vi "Nchw_CheckSize.vi"(4 "NumberOfMats":i32, 6 "MatToFit":T1, 8 "Width":i32, 9 "Height":i32, 10 "Channels":i32, 11 "Dimensions":i32) -> (3 "same":bool)   [LabVIEW 2020, in "OpenLvVision_OpenCv.lvlib"]
uses:
  OpenLvVision_OpenCv.lvlib
  TypeDef/LvDatatype.ctl
  TypeDef/MatInfo.ctl
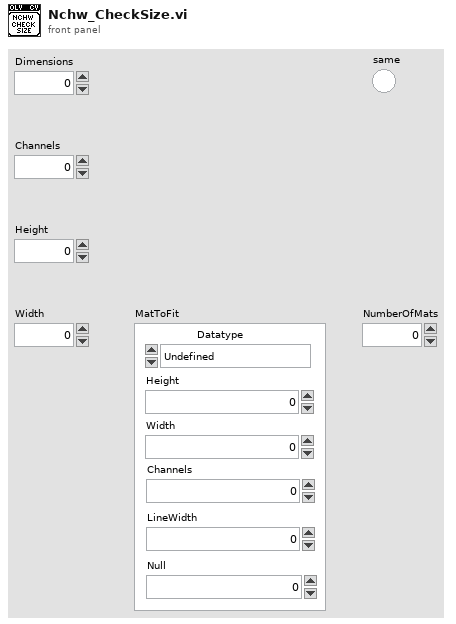
[diagram p1: front panel]
types:
  T1 = typedef "OpenLvVision_OpenCv.lvlib/MatInfo.ctl" = cluster{"Datatype":T2, "Height":i32, "Width":i32, "Channels":i32, "LineWidth":i32, "Null":u8}
  T2 = typedef "OpenLvVision_OpenCv.lvlib/LvDatatype.ctl" = enum32{"Undefined", "U8", "I8", "U16", "I16", "U32_Color", "I32", "U64_Color", "I64", "SGL", "DBL", "Complex SGL", "Complex DBL", "Array 1D U8", "Array 1D I8", "Array 1D U16", "Array 1D I16", "Array 1D U32_Color", "Array 1D I32", "Array 1D U64_Color", "Array 1D I64", "Array 1D SGL", "Array 1D DBL", "Array 1D Complex SGL", "Array 1D Complex DBL", "Array 2D U8", "Array 2D I8", "Array 2D U16", "Array 2D I16", "Array 2D U32", "Array 2D U32_Color", "Array 2D I32", "Array 2D U64", "Array 2D U64_Color", "Array 2D I64", "Array 2D SGL", "Array 2D DBL", "Array 2D Complex SGL", "Array 2D Complex DBL", "Image Mono U8", "Image Mono U16", "Image Mono I16", "Image Mono SGL", "Image Color U32", "Image Color U64", "ImageComplex Sgl", "Array1d_2dPointI32", "Array1d_2dPointSGL", "Array1d_2dPointDBL", "Array1d_3dPointI32", "Array1d_3dPointSGL", "Array1d_3dPointDBL", "Array1d_4dPointI32", "Array1d_4dPointSGL", "Array1d_4dPointDBL", "ArrayNchwU8", "ArrayNchwI8", "ArrayNchwU16", "ArrayNchwI16", "ArrayNchwU32_Color", "ArrayNchwI32", "ArrayNchwU64_Color", "ArrayNchwSgl", "ArrayNchwDbl", "ArrayNchwComplexSgl", "ArrayNchwComplexDbl"}
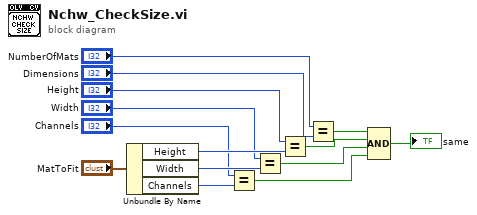
[diagram p0: block diagram]
diagram:
  n1 = Unbundle By Name("MatToFit") -> ("Height"=w13:i32, "Width"=w11:i32, "Channels"=w9:i32)
  n2 = Equal?(x="Channels", y=w9) -> (x = y?=w2:bool)
  n3 = Equal?(x="Width", y=w11) -> (x = y?=w3:bool)
  n4 = Equal?(x="Height", y=w13) -> (x = y?=w4:bool)
  n5 = Equal?(x="NumberOfMats", y="Dimensions") -> (x = y?=w5:bool)
  n6 = Compound Arithmetic op=AND(w5, w4, w3, w2) -> (→"same":bool)
